vi "PmacCoordScale.vi"(1 "Coord Number i32 (1-8) (1)":i32(knob) min=1 max=8 scale=1.0..8.0, 2 "Device Number i32 (0)":i32 min=0) -> (0 "Coordinate System Scale Cluster":T1 {"Coordinate System" min=1 max=8})   [LabVIEW 2020]
doc: "Query PMAC for the motors defined in Coord Number. The Coordinate System Scale Cluster (PmacCoordScale.ctl) contains three arrays with the motor definition, scale factor, and whether or not the motor is definined in Coord Number. The actual query is only placed if Coord Number changes from a previous call."
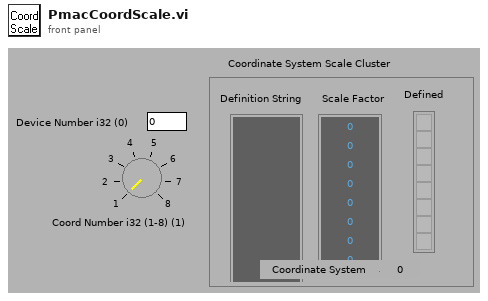
[diagram p1: front panel]
types:
  T1 = cluster{"Definition String":string[], "Scale Factor":i32[], "Defined":bool[], "Coordinate System":i32}
  T2 = cluster{string[], dbl[], bool[], "Coord Number i32 (1-8) (1) ":i32}
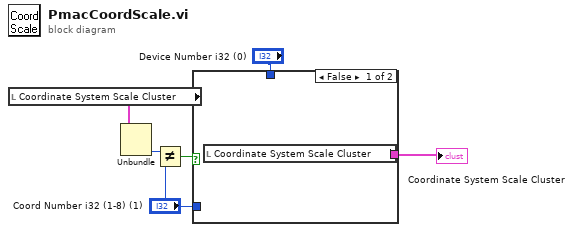
[diagram p0: block diagram]
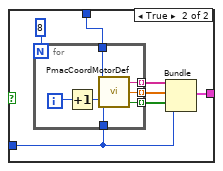
[diagram p2: hidden frame]
diagram:
  n1 = local read "Coordinate System Scale Cluster"() -> (w2:T1)
  n2 = Unbundle(w2) -> ("Coordinate System"=w1:i32)  [unwired: 3 out]
  n3 = Not Equal?(x=w1, y="Coord Number i32 (1-8) (1)") -> (x != y?=w5:bool)
  n4 = case shown="False" w5 {
    tunnel: "Device Number i32 (0)" -> [_ w10]
    tunnel: "Coord Number i32 (1-8) (1)" -> [_ w9]
    tunnel: [w7 w8] -> w3
    frame False {
      n5 = local read "Coordinate System Scale Cluster"() -> (w7:T1)
    }
    frame True {
      n6 = for {
        N: 8 -> [_]
        tunnel: [w19] -> w12 mode=indexing
        tunnel: [w18] -> w13 mode=indexing
        tunnel: [w17] -> w14 mode=indexing
        tunnel: w10 -> [w16]
        tunnel: w9 -> [w15]
        i -> [w21]
        n7 = Increment(x=w21) -> (x+1=w20:i32)
        n8 = call "PmacCoordMotorDef.vi"("Motor Number i32 (1-8) (1)"=w20, "Coord Number i32 (1-8) (1)"=w15, "Device Number i32 (0)"=w16) -> ("Coord Defined Bool (F)"=w17:bool, "Coord Scale Dbl (1.0)"=w18:dbl, "Coord Definition String"=w19:string)
      }
      n9 = Bundle(w12, w13, w14, "Coord Number i32 (1-8) (1)"=w9) -> (w8:T2)  [unwired: 1 out]
    }
  }
  "Coordinate System Scale Cluster" <- w3
